vi "校准泵控制.vi"(8 "错误输入（无错误）":errorcluster, 9 "摄氏度":u16, 10 "偏心轮":u16, 11 "枚举":enum16{"进水样", "排液", "加热", "停止"}(ring)) -> (0 "错误输出":errorcluster)   [LabVIEW 2016, in "斯坦道CODMn新电路板.lvlib"]
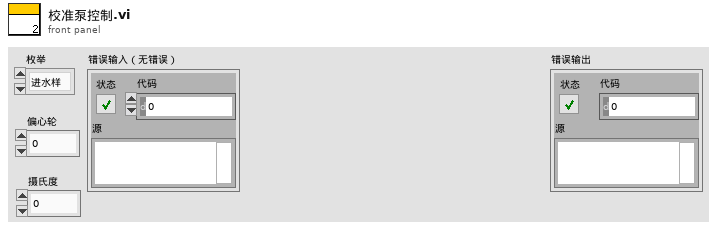
[diagram p1: front panel]
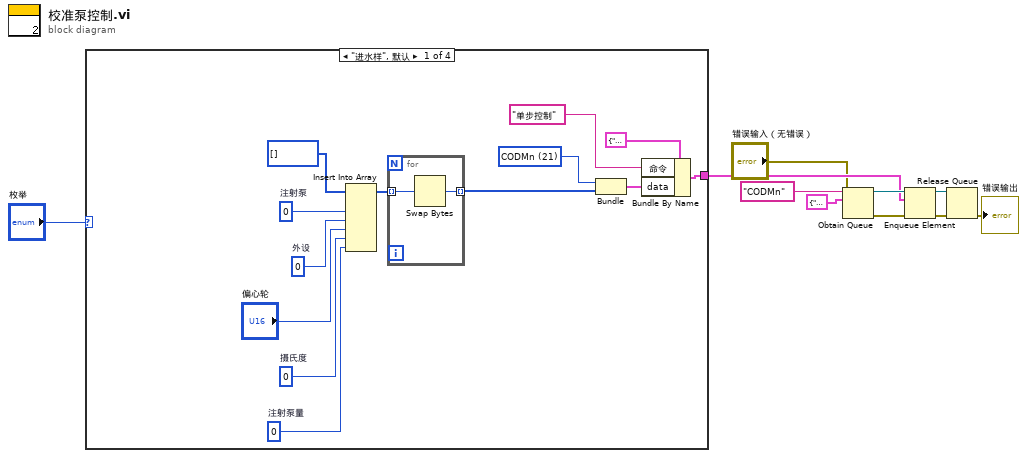
[diagram p0: block diagram]
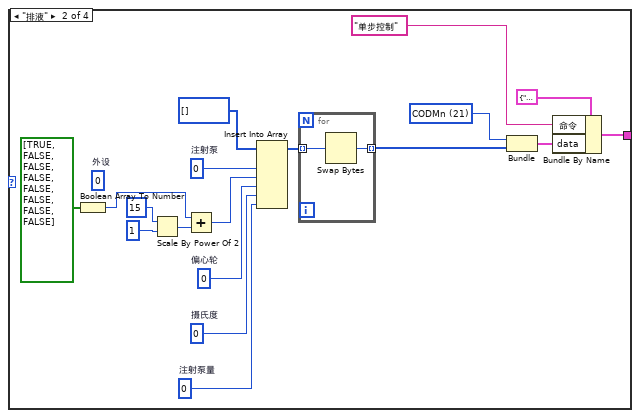
[diagram p2: hidden frame]
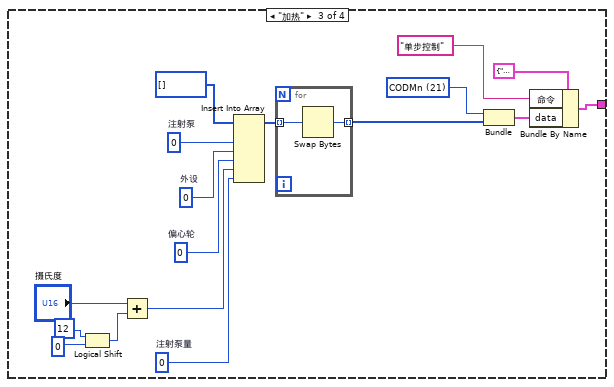
[diagram p3: hidden frame]
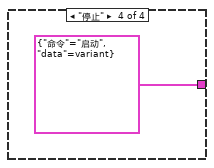
[diagram p4: hidden frame]
diagram:
  n1 = case shown="\"进水样\", 默认" "枚举" {
    tunnel: [w11 w32 w51 cluster{"命令":string, "data":variant} {"命令"="启动", "data"=variant(cluster{"站号":u16, "控制命令":u16[]} {"站号"=21, "控制命令"=[2816]})} ("启动命令")] -> w3
    frame "进水样", Default {
      w16 = u16 21 items=["CODMn"=21, "总磷"=1, "氨氮"=3] ("站号")
      w20 = u16 0  # 注射泵量
      w19 = u16 0  # 摄氏度
      w21 = u16 0  # 外设
      w22 = u16 0  # 注射泵
      n2 = Insert Into Array(array=u16[] [] ("数组"), new element #1=w22, new element #2=w21, new element #3="偏心轮", new element #4=w19, new element #5=w20) -> (w18:u16[])  [unwired: 1 in]
      n3 = for {
        tunnel: w18 -> [w25] mode=indexing
        tunnel: [w24] -> w13 mode=indexing
        n4 = Swap Bytes(anything=w25) -> (byte swapped=w24:u16)
      }
      n5 = Bundle("站号"=w16, w13) -> (w15:cluster{"站号":u16, u16[]})  [unwired: 1 in]
      n6 = Bundle By Name(cluster=cluster{"命令":string, "data":variant} {"命令"="", "data"=variant} ("元素"), "命令"="单步控制", "data"=w15) -> (w11:cluster{"命令":string, "data":variant})
    }
    frame "排液" {
      w37 = u16 21 items=["CODMn"=21, "总磷"=1, "氨氮"=3] ("站号")
      w41 = u16 0  # 注射泵量
      w40 = u16 0  # 摄氏度
      w38 = u16 0  # 偏心轮
      (unwired) u16 0  # 外设
      w42 = u16 0  # 注射泵
      n7 = Boolean Array To Number ("布尔数组至数值转换")(Boolean array=bool[] [TRUE, FALSE, FALSE, FALSE, FALSE, FALSE, FALSE, FALSE] ("添加的数组")) -> (number=w31:u16)
      n8 = Scale By Power Of 2(n=i16 15, x=u16 1 ("y")) -> (x*2^n=w30:u16)
      n9 = Add(x=w31, y=w30) -> (x+y=w26:u16)
      n10 = Insert Into Array(array=u16[] [] ("数组"), new element #1=w42, new element #2=w26, new element #3=w38, new element #4=w40, new element #5=w41) -> (w39:u16[])  [unwired: 1 in]
      n11 = for {
        tunnel: w39 -> [w45] mode=indexing
        tunnel: [w44] -> w34 mode=indexing
        n12 = Swap Bytes(anything=w45) -> (byte swapped=w44:u16)
      }
      n13 = Bundle("站号"=w37, w34) -> (w36:cluster{"站号":u16, u16[]})  [unwired: 1 in]
      n14 = Bundle By Name(cluster=cluster{"命令":string, "data":variant} {"命令"="", "data"=variant} ("元素"), "命令"="单步控制", "data"=w36) -> (w32:cluster{"命令":string, "data":variant})
    }
    frame "加热" {
      w56 = u16 21 items=["CODMn"=21, "总磷"=1, "氨氮"=3] ("站号")
      w59 = u16 0  # 注射泵量
      w57 = u16 0  # 偏心轮
      w60 = u16 0  # 外设
      w61 = u16 0  # 注射泵
      n15 = Logical Shift(y=i16 12, x=i16 0) -> (x << y=w49:i16)
      n16 = Add(x="摄氏度", y=w49) -> (x+y=w46:u16)
      n17 = Insert Into Array(array=u16[] [] ("数组"), new element #1=w61, new element #2=w60, new element #3=w57, new element #4=w46, new element #5=w59) -> (w58:u16[])  [unwired: 1 in]
      n18 = for {
        tunnel: w58 -> [w64] mode=indexing
        tunnel: [w63] -> w53 mode=indexing
        n19 = Swap Bytes(anything=w64) -> (byte swapped=w63:u16)
      }
      n20 = Bundle("站号"=w56, w53) -> (w55:cluster{"站号":u16, u16[]})  [unwired: 1 in]
      n21 = Bundle By Name(cluster=cluster{"命令":string, "data":variant} {"命令"="", "data"=variant} ("元素"), "命令"="单步控制", "data"=w55) -> (w51:cluster{"命令":string, "data":variant})
    }
    frame "停止" {
    }
  }
  n22 = Obtain Queue(name (unnamed)="CODMn" ("名称（未命名）"), element data type=cluster{"命令":string, "data":variant} {"命令"="", "data"=variant}, error in (no error)="错误输入（无错误）") -> (queue out=w8:refnum<queue>, error out=w7:errorcluster)  [unwired: 2 in, 1 out]
  n23 = Enqueue Element(queue=w8, element=w3, error in (no error)=w7) -> (queue out=w6:refnum<queue>, error out=w5:errorcluster)  [unwired: 1 in, 1 out]
  n24 = Release Queue(queue=w6, error in (no error)=w5) -> (error out=→"错误输出":errorcluster)  [unwired: 1 in, 2 out]
